vi "secondaire.vi"() -> ()   [LabVIEW 2018]
uses:
  Global 1.vi
panel:
  in  "stop":bool
  in  "Code secret à changer":i16
  in  "Maximum de tentatives à changer":i32
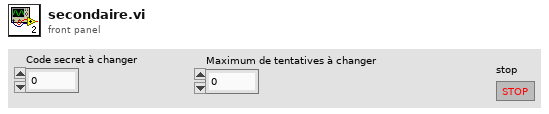
[diagram p1: front panel]
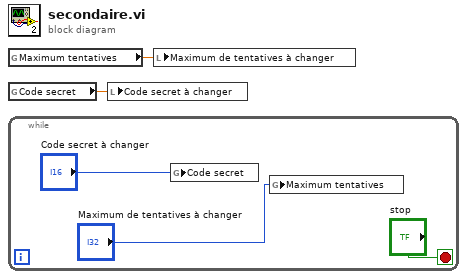
[diagram p0: block diagram]
diagram:
  n1 = global read "Global 1.vi" "Maximum tentatives"() -> (w1:dbl)
  n2 = global read "Global 1.vi" "Code secret"() -> (w2:dbl)
  n3 = while {
    stop <- "stop" stop-if-true
    n4 = global write "Global 1.vi" "Code secret"("Code secret à changer") -> ()
    n5 = global write "Global 1.vi" "Maximum tentatives"("Maximum de tentatives à changer") -> ()
  }
  n6 = local write "Code secret à changer"(w2) -> ()
  n7 = local write "Maximum de tentatives à changer"(w1) -> ()
